vi "Next Step.vi"(0 "Zone Setup Array in":cluster{"Zone Selector":string, "Timing":dbl}[](array[cluster]), 1 "Run Selector Reference":refnum<vi>, 2 "Controller Status":string, 5 "Step Status In":string="New Step", 7 "Step In":i32, 9 "Time completed?":bool=TRUE, 11 "error in":errorcluster) -> (4 "Step Status Out":string, 6 "Step Out":i32, 8 "Machine State":T1, 15 "error out":errorcluster)   [LabVIEW 2020]
doc: "This VI determine the next step based on the simulation controls and the current step status (completed or pending)."
uses:
  Machine States.ctl
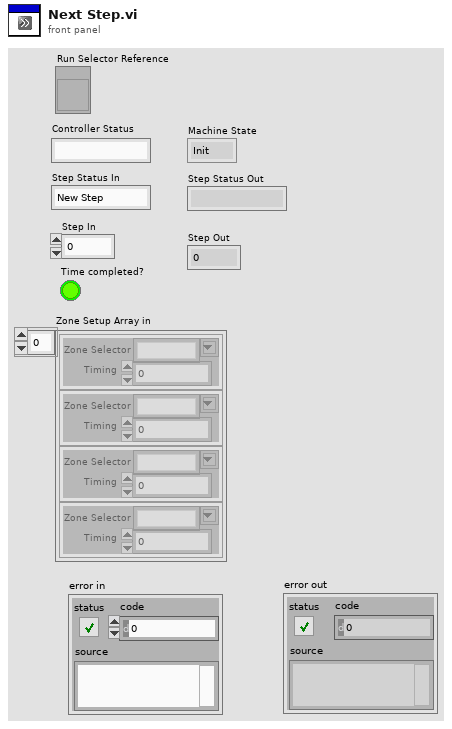
[diagram p1: front panel]
types:
  T1 = typedef "Machine States.ctl" = enum16{"Init", "Setup", "Start", "Stop", "Wait To Start", "Low Water Pressure", "Rain"}
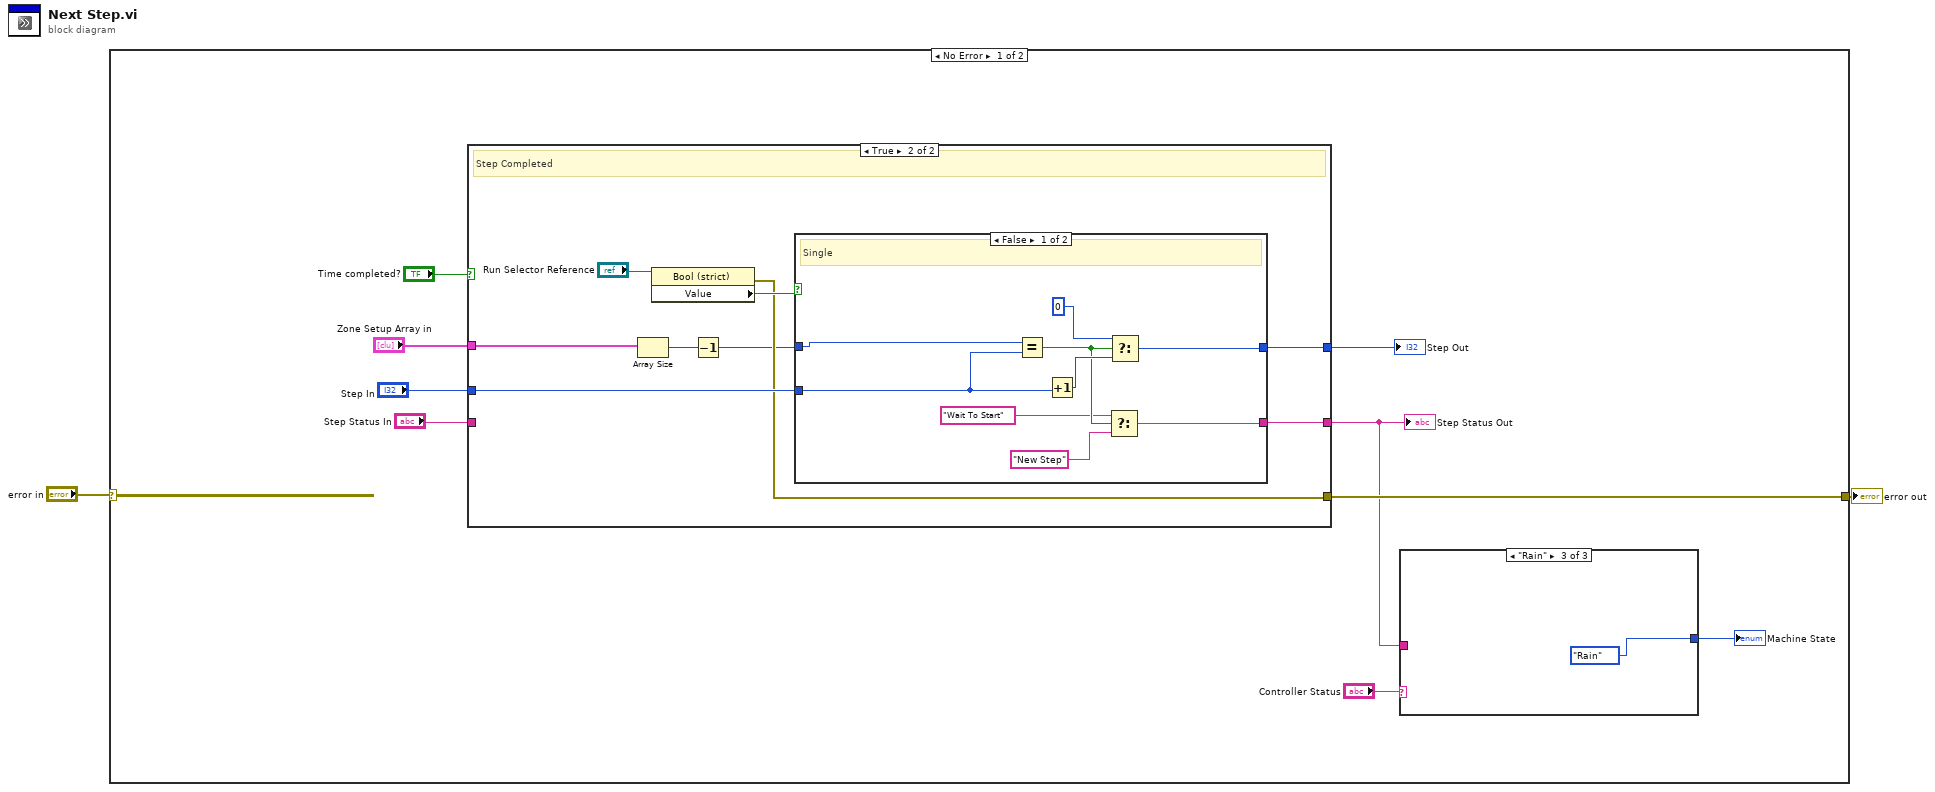
[diagram p0: block diagram]
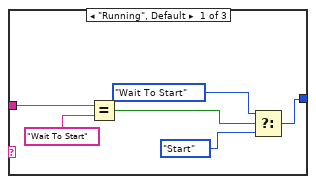
[diagram p2: hidden frame]
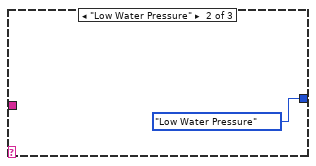
[diagram p3: hidden frame]
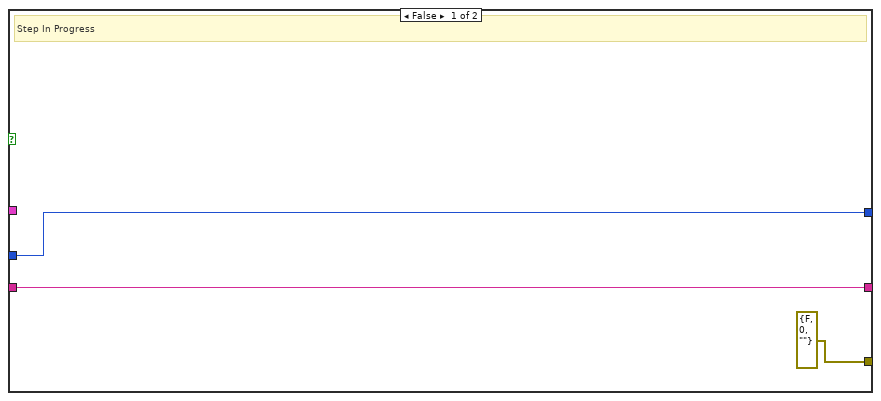
[diagram p4: hidden frame]
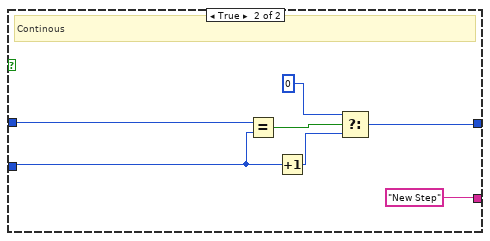
[diagram p5: hidden frame]
diagram:
  n1 = case shown="No Error" "error in" {
    selector: "error in" -> [_ w48]
    tunnel: [w6 w48] -> w1
    frame No Error {
      n2 = case shown="True" "Time completed?" {
        tunnel: [w22 w29] -> w10
        tunnel: [w21 w28] -> w3
        tunnel: "Zone Setup Array in" -> [_ w25]
        tunnel: "Step In" -> [w22 w27]
        tunnel: "Step Status In" -> [w21 _]
        tunnel: [errorcluster {"status"=FALSE, "code"=0, "source"=""} ("error out") w26] -> w6
        frame False {
          # "Step In Progress"
        }
        frame True {
          # "Step Completed"
          n3 = Array Size(array=w25) -> (size(s)=w24:i32)
          n4 = property class="Bool (strict)"(reference="Run Selector Reference") -> (error out=w26:errorcluster, "Value"=w30:bool)  [unwired: 1 in, 1 out]
          n5 = Decrement(x=w24) -> (x-1=w23:i32)
          n6 = case shown="False" w30 {
            tunnel: [w38 w44] -> w29
            tunnel: [w34 "New Step" ("f")] -> w28
            tunnel: w27 -> [w33 w43]
            tunnel: w23 -> [w32 w41]
            frame False {
              # "Single"
              n7 = Equal?(x=w32, y=w33) -> (x = y?=w37:bool)
              n8 = Increment(x=w33) -> (x+1=w39:i32)
              n9 = Select(t="Wait To Start", s=w37, f="New Step") -> (s? t:f=w34:string)
              n10 = Select(t=0 ("Step"), s=w37, f=w39) -> (s? t:f=w38:i32)
            }
            frame True {
              # "Continous"
              n11 = Equal?(x=w41, y=w43) -> (x = y?=w45:bool)
              n12 = Increment(x=w43) -> (x+1=w46:i32)
              n13 = Select(t=0 ("Step"), s=w45, f=w46) -> (s? t:f=w44:i32)
            }
          }
        }
      }
      "Step Out" <- w10
      "Step Status Out" <- w3
      n14 = case shown="\"Rain\"" "Controller Status" {
        tunnel: [w12 Machine_States."Low Water Pressure" ("f") Machine_States."Rain" ("f")] -> w4
        tunnel: w3 -> [w13 _ _]
        frame "Running", Default {
          n15 = Equal?(x=w13, y="Wait To Start") -> (x = y?=w17:bool)
          n16 = Select(t=Machine_States."Wait To Start" ("Enum"), s=w17, f=Machine_States."Start") -> (s? t:f=w12:T1)
        }
        frame "Low Water Pressure" {
        }
        frame "Rain" {
        }
      }
      "Machine State" <- w4
    }
    frame Error {
    }
  }
  "error out" <- w1
